vi "Refresh.vi"(8 "error in (no error)":errorcluster, 11 "InsertionPalettePanel in":refnum<class "InsertionPalettePanel.lvclass">) -> (0 "error out":errorcluster, 3 "InsertionPalettePanel out":refnum<class "InsertionPalettePanel.lvclass">)   [LabVIEW 2020, in "TSnax UI.lvlib" / "InsertionPalettePanel.lvclass"]
uses:
  InsertionPalettePanel.lvclass
  InsertionPalettePanel.lvclass/InsertionPalettePanel.ctl
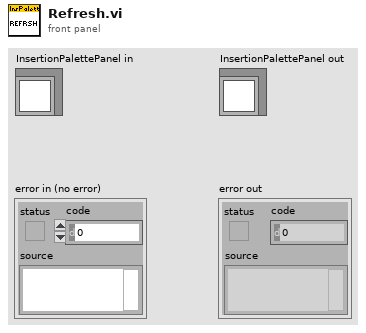
[diagram p1: front panel]
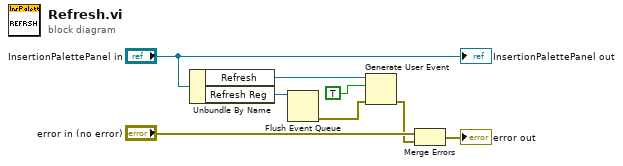
[diagram p0: block diagram]
diagram:
  n1 = Unbundle By Name("InsertionPalettePanel in") -> ("Refresh"=w5:refnum<user-event>, "Refresh Reg"=w6:refnum<event-registration>)
  n2 = Flush Event Queue(0:w6) -> (11:w4:errorcluster)  [unwired: 5 in, 2 out]
  n3 = Generate User Event(user event=w5, event data cluster=TRUE ("event data"), error in=w4) -> (error out=w1:errorcluster)  [unwired: 1 in, 1 out]
  n4 = Merge Errors("error in (no error)", w1) -> (→"error out":errorcluster)
  "InsertionPalettePanel out" <- "InsertionPalettePanel in"
